vi "SetupZSpan.vi"(8 "error in (no error)":errorcluster, 10 "Center Freq (Hz)":dbl=13250000000.0 format="%#.6g", 11 "SigGen_MXG.In":refnum<class "SigGen_MXG.lvclass">) -> (0 "error out":errorcluster, 3 "SigGen_MXG.Out":refnum<class "SigGen_MXG.lvclass">)   [LabVIEW 2014, in "SigGen_MXG.lvclass"]
uses:
  SigGen_MXG.lvclass
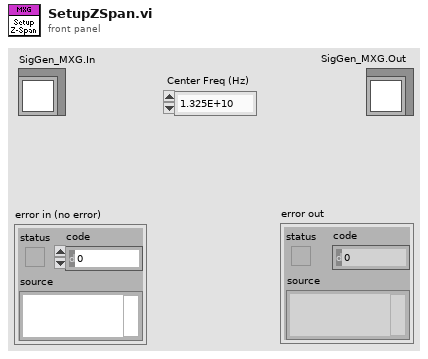
[diagram p1: front panel]
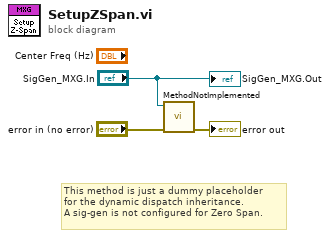
[diagram p0: block diagram]
diagram:
  # "This method is just a dummy placeholder\nfor the dynamic dispatch inheritance.\nA sig-gen is not configured for Zero Span."
  n1 = call "MethodNotImplemented.vi"("error in (no error)"="error in (no error)", "LabVIEW Object In"="SigGen_MXG.In") -> ("error out"=→"error out":errorcluster)  [unwired: 9 in]
  "SigGen_MXG.Out" <- "SigGen_MXG.In"
